vi "导出文件流程.vi"(0 "刷新错误?":refnum<vi>, 1 "刷新信号-引用":refnum<vi>, 2 "XY图更新错误?":refnum<vi>, 3 "XY图-引用":refnum<vi>, 6 "错误输入":errorcluster, 7 "查询界面VI-引用":refnum<vi>, 8 "累积记录-引用":refnum<vi>, 9 "设备清单-引用":refnum<vi>, 10 "设备列表-引用":refnum<vi>, 11 "导出条件":T2) -> (4 "错误输出":errorcluster)   [LabVIEW 2017]
uses:
  e6222c88-c07e-4ecc-8f52-69902710a8a5.vi
  642c5d25-862a-469e-85c1-2600a8577a38.vi
  <vilib>/Utility/file.llb/Write Delimited Spreadsheet (string).vi
panel:
  in  "刷新次数":i32
  in  "原界面模式":T1
  out "提示语":string
  # "导出记录执行中......"
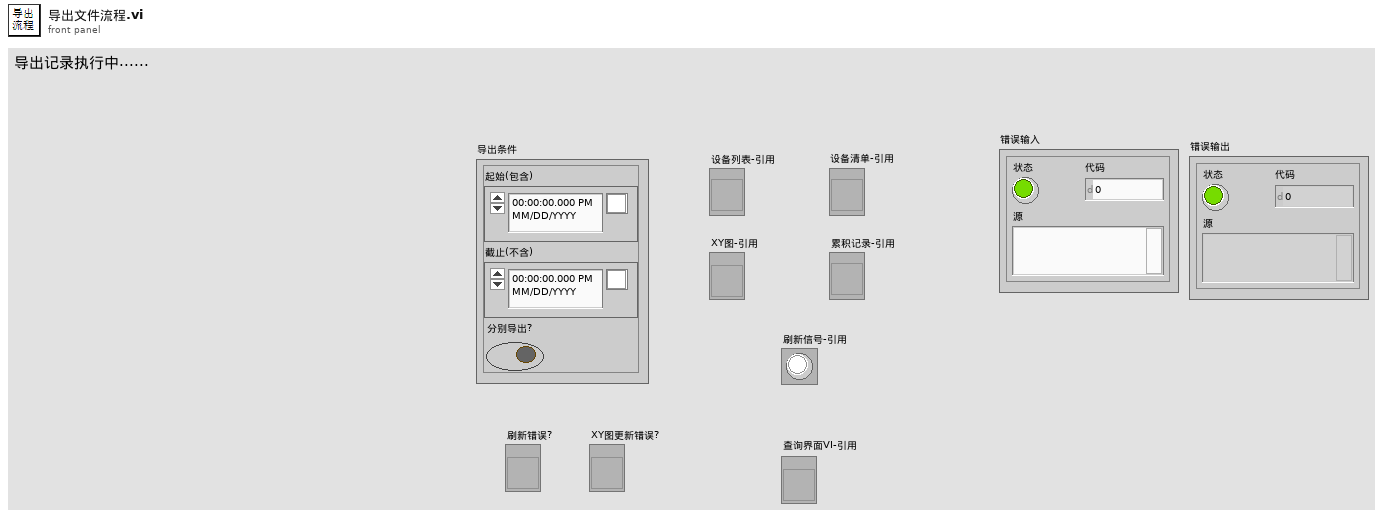
[diagram p1: front panel]
types:
  T1 = typedef "枚举-顶层框架功能模式.ctl" = enum16{"管理模式", "监测模式", "浏览模式"}
  T2 = typedef "文件导出条件.ctl" = cluster{"起始(包含)":timestamp, "截止(不含)":timestamp, "分别导出?":bool}
  T3 = typedef "定时配置.ctl" = cluster{"定时模式":enum16{"绝对时间", "相对时间"}, "单位":enum16{"年", "月", "日", "时", "分"}, "间隔":u8, "目标时刻":timestamp}
  T4 = enum32{"Invalid", "Standard", "Closed", "Hidden", "Minimized", "Maximized"}
  T5 = typedef "探测器信息.ctl" = cluster{"网络地址":string, "名称":string, "备注":string, "累积剂量":dbl, "累积限值":dbl, "硬件剂量率限值":T6, "剂量率限值1":dbl, "剂量率限值2":dbl, "报警方式":T7}
  T6 = typedef "探头剂量率限值选择.ctl" = enum16{"一级限值", "二级限值"}
  T7 = typedef "报警方式选择.ctl" = enum16{"常报警", "自动静音", "手动静音"}
  T8 = typedef "单条累积记录.ctl" = cluster{"起始时间":timestamp, "结束时间":timestamp, "累积剂量":dbl}
  T9 = typedef "通用报警记录.ctl" = cluster{"探头状态":T10, "探头地址与信息":T5, "缓存绘图数据":T11, "平均值":dbl, "报警时长":cluster{"分":u16, "秒":u16}, "结论":string}
  T10 = typedef "探头状态.ctl" = enum16{"正常", "离线", "禁用", "一级报警", "二级报警", "累积报警"}
  T11 = typedef "缓存数据.ctl" = cluster{"时间":timestamp[], "数值":dbl[], "压缩等级数量":i32[], "最大值":cluster{"时间":timestamp, "数值":dbl}, "起始点":cluster{"时间":timestamp, "数值":dbl}, "容量限值":i32, "报警累积":dbl}
  T12 = cluster{"累积曲线数据":T8[], "累积列表内容":string[], "匹配的报警数据":cluster{"名称":string, "路径":path, "内容":string, "报警记录":T9}[]}[]
  T13 = typedef "imagedata.ctl" = cluster{"image type":i32, "image depth":i32, "image":u8[], "mask":u8[], "colors":u32[], "Rectangle":cluster{"left":i16, "top":i16, "right":i16, "bottom":i16}}
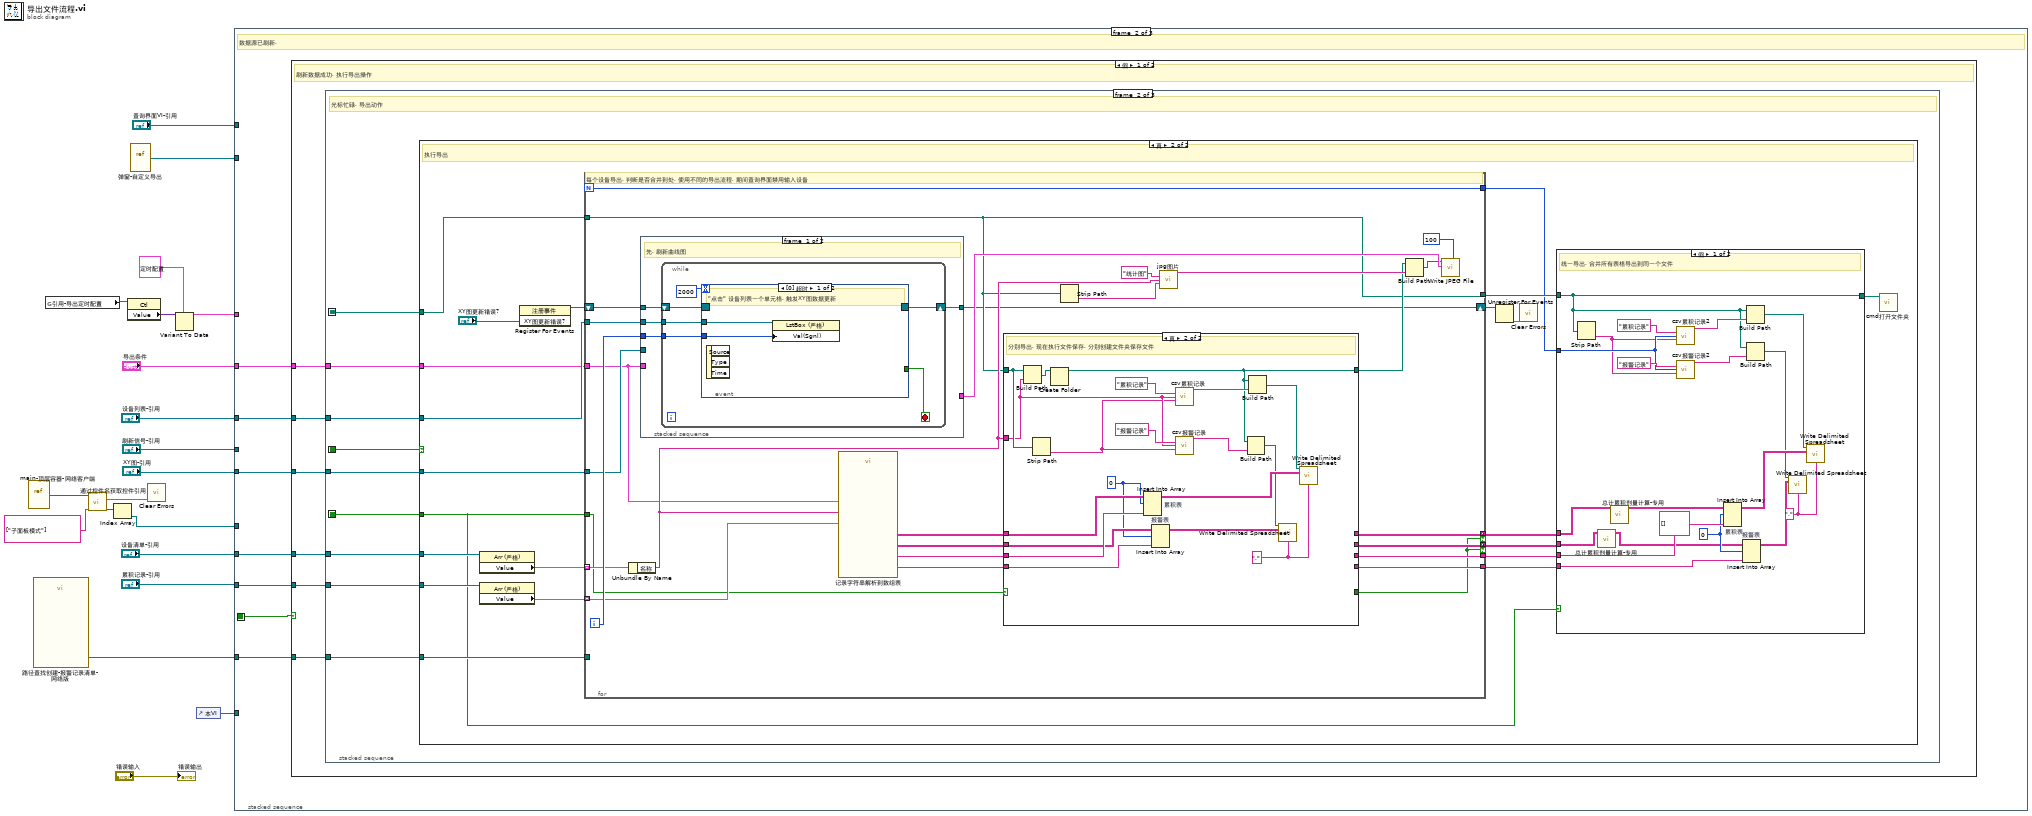
[diagram p0: block diagram]
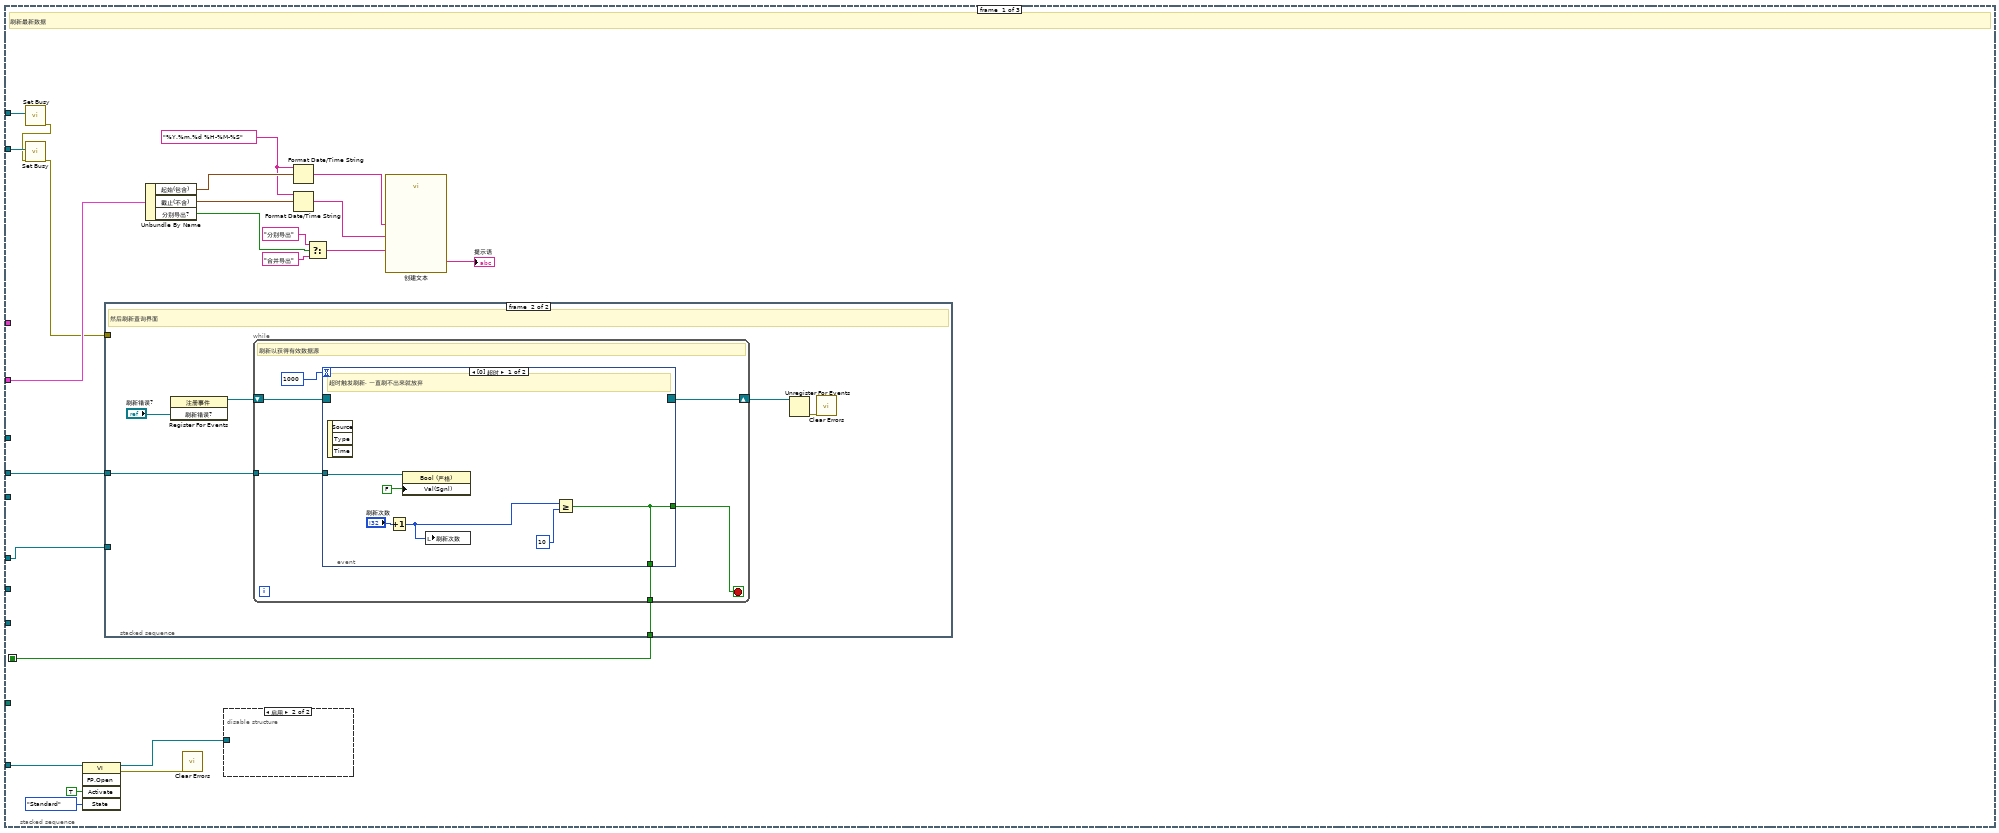
[diagram p2: hidden frame]
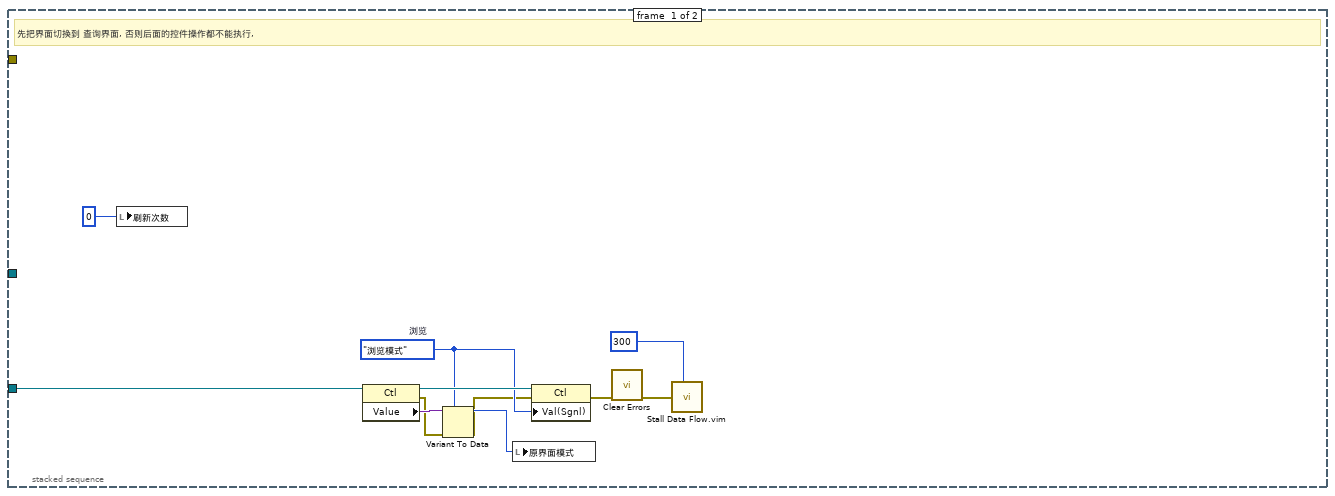
[diagram p3: hidden frame]
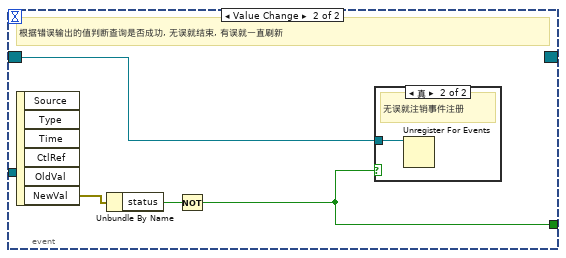
[diagram p4: hidden frame]
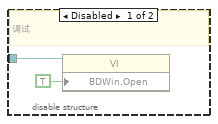
[diagram p6: hidden frame]
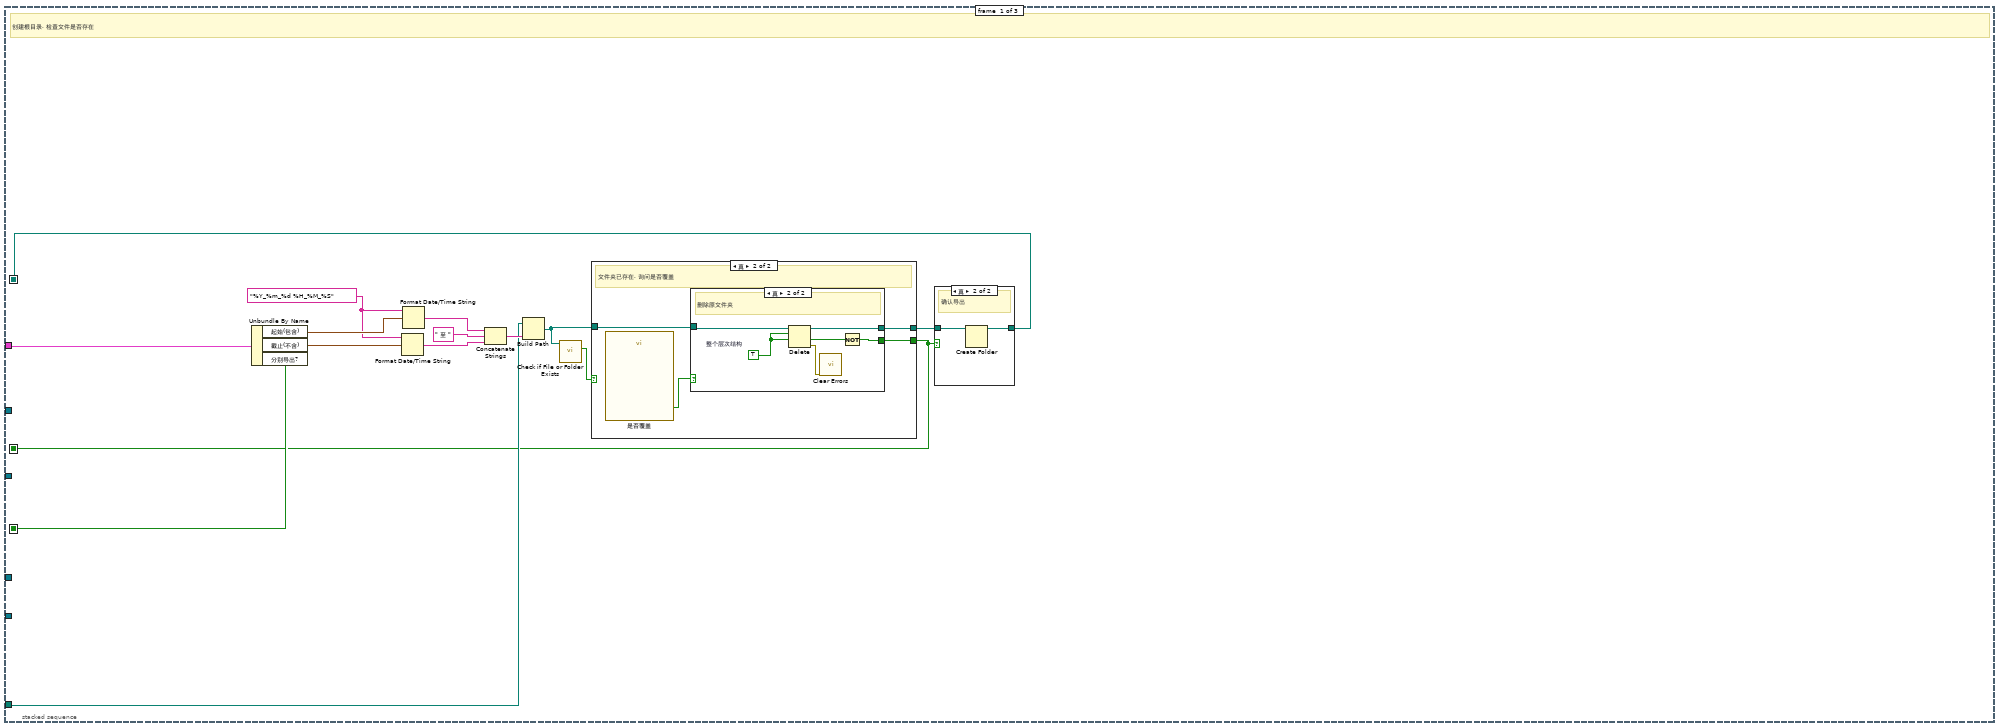
[diagram p7: hidden frame]
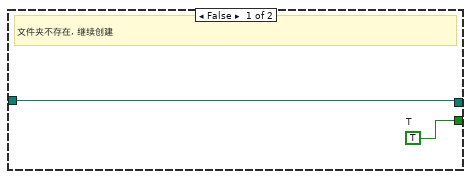
[diagram p8: hidden frame]
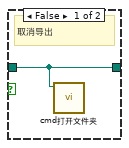
[diagram p10: hidden frame]
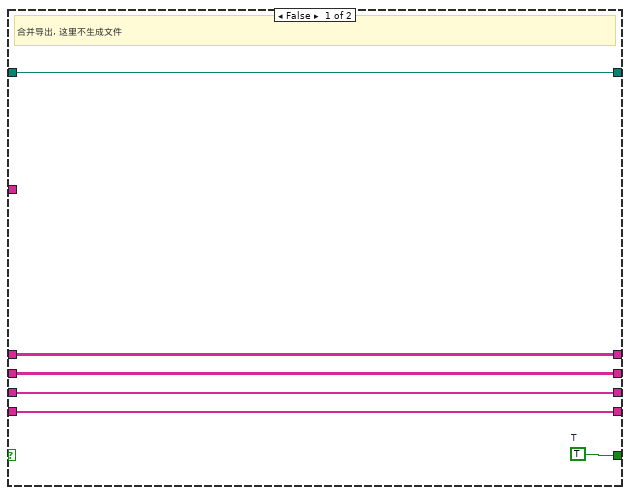
[diagram p13: hidden frame]
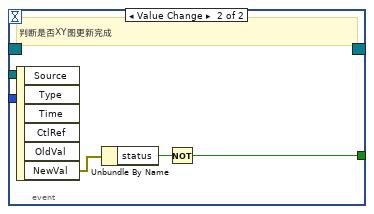
[diagram p14: hidden frame]
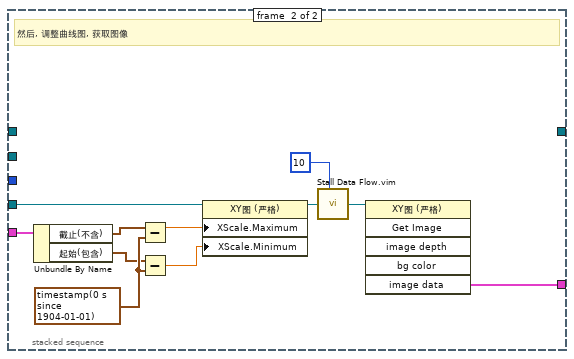
[diagram p15: hidden frame]
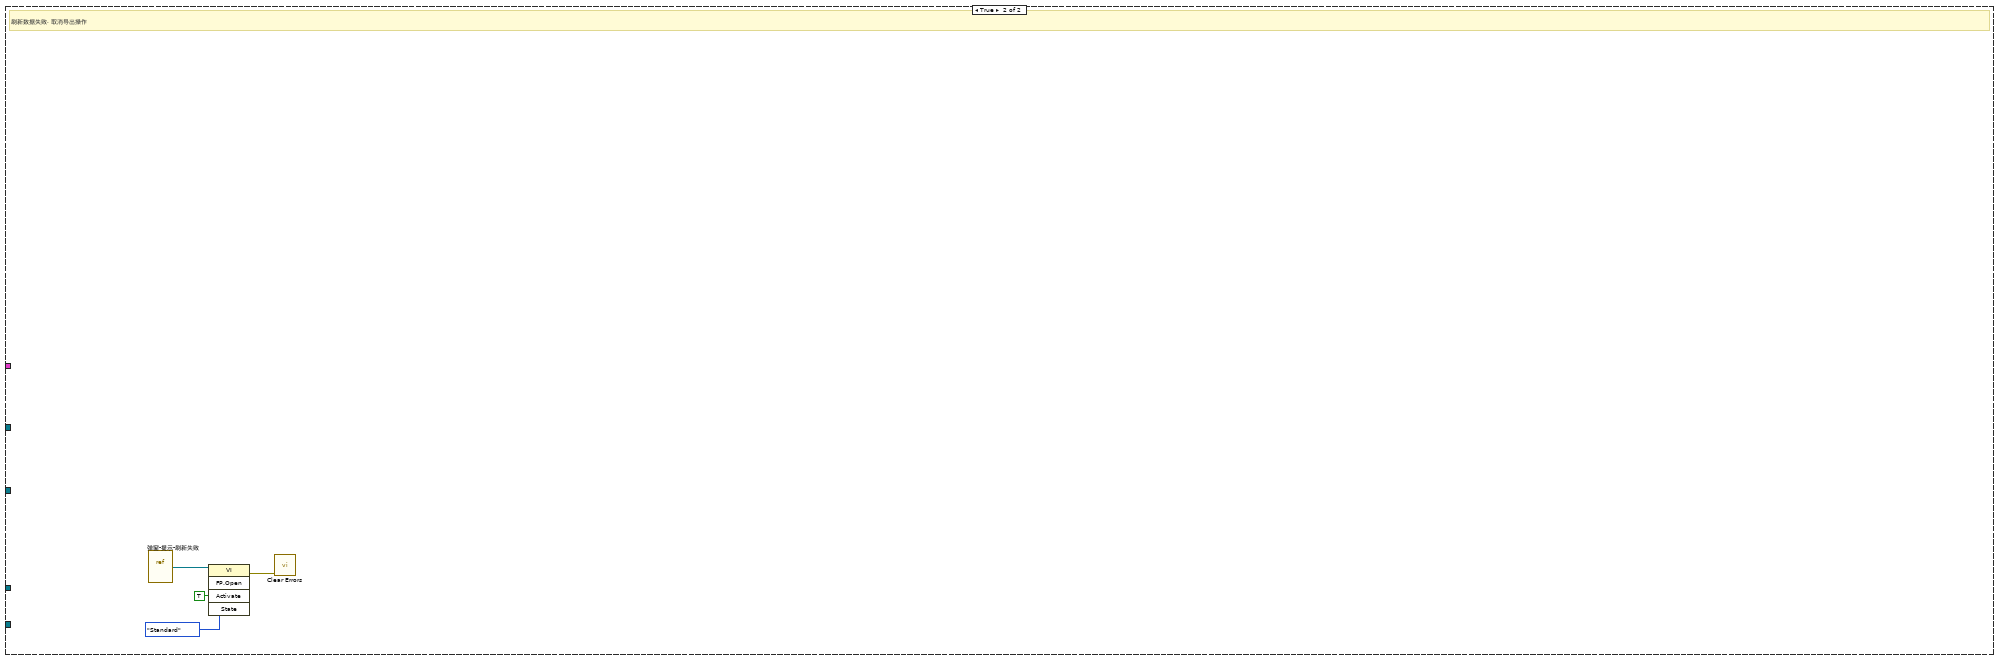
[diagram p17: hidden frame]
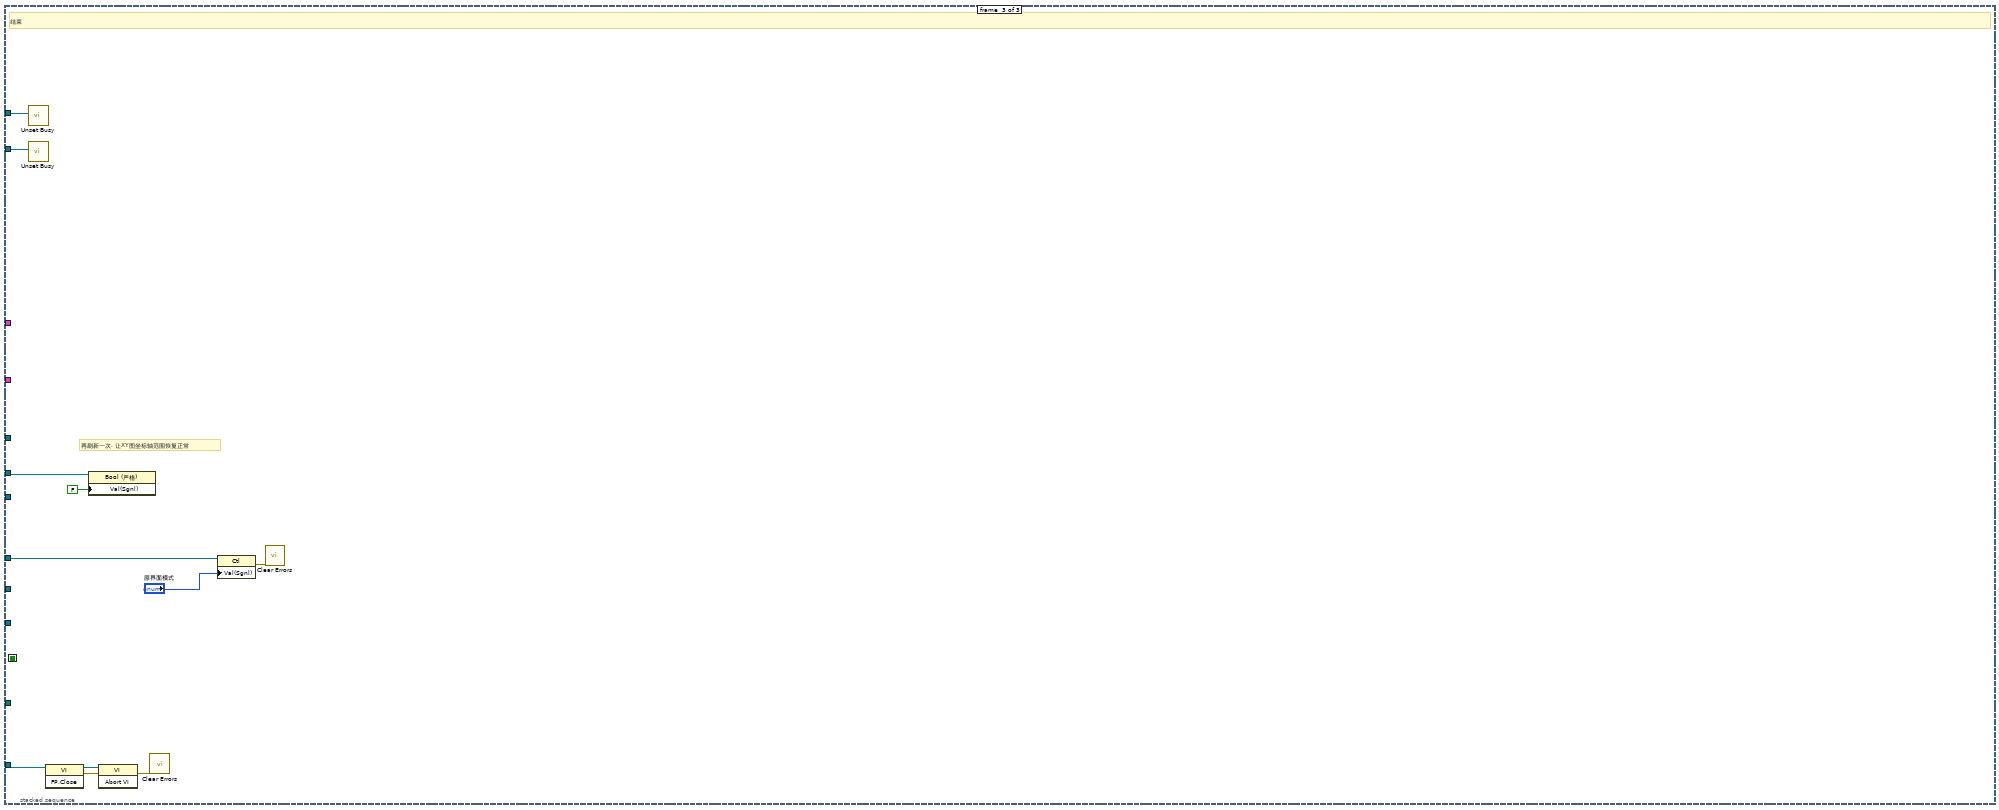
[diagram p18: hidden frame]
diagram:
  n1 = vi-ref "main-顶层容器-网络客户端.vi"() -> (w6:refnum<vi>)
  n2 = call "路径查找创建-报警记录清单-网络版.vi"() -> ("导出记录"=w11:path)  [unwired: 2 in, 13 out]
  n3 = global read "全局变量-35点监测.vi" "引用-导出定时配置"() -> (w15:refnum<vi>)
  n4 = call "通过控件名获取控件引用.vi"("控件名数组"=string[] ["子面板模式"], "VI引用"=w6) -> ("控件引用输出"=w5:refnum<vi>[], "错误输出"=w2:errorcluster)  [unwired: 7 in, 1 out]
  n5 = Index Array(array=w5) -> (element=w3:refnum<vi>)  [unwired: 1 in]
  n6 = property class="Ctl"(reference=w15) -> ("Value"=w14:variant)  [unwired: 1 in, 2 out]
  n7 = vi-ref "弹窗-自定义导出.vi"() -> (w1:refnum<vi>)
  n8 = call <vilib>:"Clear Errors.vi"("error in (no error)"=w2) -> ()  [unwired: 5 in, 2 out]
  n9 = Variant To Data(type=T3 {"定时模式"=enum."绝对时间", "单位"=enum."年", "间隔"=0, "目标时刻"=timestamp(0 s since 1904-01-01)} ("定时配置"), Variant=w14) -> (data=w12:T3)  [unwired: 1 in, 1 out]
  n10 = control-ref of="本VI"() -> (w8:refnum<vi>)
  n11 = stacked-sequence {
    seq-local: [w26 _ _] -> [_ w80 _]
    tunnel: "设备列表-引用" -> [_ w84 _]
    tunnel: "刷新信号-引用" -> [w43 _ w262]
    tunnel: "XY图-引用" -> [_ w85 _]
    tunnel: "设备清单-引用" -> [_ w86 _]
    tunnel: "累积记录-引用" -> [_ w83 _]
    tunnel: "导出条件" -> [w42 w82 _]
    tunnel: w12 -> [_ _ _]
    tunnel: w11 -> [_ w81 _]
    tunnel: w8 -> [w31 _ w267]
    tunnel: "查询界面VI-引用" -> [w25 _ w259]
    tunnel: w3 -> [w24 _ w258]
    tunnel: w1 -> [w23 _ w257]
    frame #0 {
      w39 = "%Y.%m.%d %H-%M-%S" ("时间格式字符串(%c)")
      # "刷新最新数据"
      n12 = call <vilib>:"Set Busy.vi"("VI reference (current VI)"=w25) -> ("error out"=w22:errorcluster)  [unwired: 9 in, 1 out]
      n13 = call <vilib>:"Set Busy.vi"("error in (no error)"=w22, "VI reference (current VI)"=w23) -> ("error out"=w21:errorcluster)  [unwired: 8 in, 1 out]
      n14 = invoke class="VI" method="FP.Open"(reference=w31, "Activate"=TRUE ("激活？"), "State"=T4."Standard" ("状态")) -> (reference out=w27:refnum<vi>, error out=w28:errorcluster)  [unwired: 2 in, 3 out]
      n15 = stacked-sequence {
        tunnel: w43 -> [_ w57]
        tunnel: [_ w55] -> w26
        tunnel: w21 -> [_ _]
        tunnel: w24 -> [w44 _]
        frame #0 {
          w51 = 枚举-顶层框架功能模式."浏览模式"  # 浏览
          # "先把界面切换到 查询界面, 否则后面的控件操作都不能执行,"
          n16 = local write "刷新次数"(0 ("数值输入控件")) -> ()
          n17 = property class="Ctl"(reference=w44) -> (reference out=w53:refnum<vi>, error out=w47:errorcluster, "Value"=w52:variant)  [unwired: 1 in]
          n18 = Variant To Data(error in=w47, type=w51, Variant=w52) -> (data=w50:T1, error out=w46:errorcluster)
          n19 = local write "原界面模式"(w50) -> ()
          n20 = property class="Ctl"(reference=w53, error in=w46, "Val(Sgnl)"=w51) -> (error out=w54:errorcluster)  [unwired: 1 out]
          n21 = call <vilib>:"Clear Errors.vi"("error in (no error)"=w54) -> ("error out"=w49:errorcluster)  [unwired: 5 in, 1 out]
          n22 = call "Stall Data Flow.vim"("value in"=w49, "milliseconds to wait"=u32 300) -> ()  [unwired: 2 out]
        }
        frame #1 {
          # "然后刷新查询界面"
          n23 = register-events("刷新错误?") -> (reference out=w59:refnum<event-registration>)  [unwired: 2 in, 1 out]
          n24 = while {
            tunnel: w57 -> [w63]
            shift-right: [w62] -> w56
            shift-left: w59 -> [w66]
            tunnel: [w61] -> w55
            stop <- w64 stop-if-true
            # "刷新以获得有效数据源"
            n25 = event shown="[0] 超时" {
              selector: w66 -> [_ w74]
              dyn-events: [_ _] -> w62
              timeout: 1000 -> [_ _]
              tunnel: [w69 w73] -> w64
              tunnel: w63 -> [w72 _]
              tunnel: [w69 _] -> w61
              event Timeout {
                # "超时触发刷新, 一直刷不出来就放弃"
                n26 = event-data() -> ()  [unwired: 1 in, 3 out]
                n27 = Increment(x="刷新次数") -> (x+1=w67:i32)
                n28 = property class="Bool (严格)"(reference=w72, "Val(Sgnl)"=FALSE) -> ()  [unwired: 1 in, 2 out]
                n29 = local write "刷新次数"(w67) -> ()
                n30 = Greater Or Equal?(x=w67, y=10) -> (x >= y?=w69:bool)
              }
              event Value Change {
                # "根据错误输出的值判断查询是否成功, 无误就结束, 有误就一直刷新"
                n31 = event-data() -> ("NewVal"=w76:errorcluster)  [unwired: 1 in, 5 out]
                n32 = Unbundle By Name(w76) -> ("status"=w75:bool)
                n33 = Not(x=w75) -> (.not. x?=w73:bool)
                n34 = case shown="真" w73 {
                  tunnel: w74 -> [_ w77]
                  frame False {
                  }
                  frame True {
                    # "无误就注销事件注册"
                    n35 = Unregister For Events(event registration refnum=w77) -> ()  [unwired: 1 in, 1 out]
                  }
                }
              }
            }
          }
          n36 = Unregister For Events(event registration refnum=w56) -> (error out=w58:errorcluster)  [unwired: 1 in]
          n37 = call <vilib>:"Clear Errors.vi"("error in (no error)"=w58) -> ()  [unwired: 5 in, 2 out]
        }
      }
      n38 = Unbundle By Name(w42) -> ("起始(包含)"=w41:timestamp, "截止(不含)"=w40:timestamp, "分别导出?"=w34:bool)
      n39 = call <vilib>:"Clear Errors.vi"("error in (no error)"=w28) -> ()  [unwired: 5 in, 2 out]
      n40 = disable-structure shown="启用" {
        disable-tunnel: w27 -> [w78 _]
        frame Disabled {
          # "调试"
          n41 = property class="VI"(reference=w78, "BDWin.Open"=TRUE ("程序框图窗口:打开")) -> ()  [unwired: 1 in, 2 out]
        }
        frame Enabled {
        }
      }
      n42 = Format Date/Time String(time format string (%c)=w39, seconds (now)=w40) -> (date/time string=w37:string)  [unwired: 1 in]
      n43 = Format Date/Time String(time format string (%c)=w39, seconds (now)=w41) -> (date/time string=w38:string)  [unwired: 1 in]
      n44 = Select(t="分别导出", s=w34, f="合并导出") -> (s? t:f=w33:string)
      n45 = call "创建文本"("起始"=w38, "截止"=w37, "导出模式"=w33) -> ("Result"=→"提示语":string)  [unwired: 11 in, 1 out]
    }
    frame #1 {
      # "数据源已刷新,"
      n46 = case shown="假" w80 {
        tunnel: w86 -> [w92 _]
        tunnel: w85 -> [w91 _]
        tunnel: w84 -> [w90 _]
        tunnel: w83 -> [w89 _]
        tunnel: w82 -> [w88 _]
        tunnel: w81 -> [w87 _]
        frame False {
          # "刷新数据成功, 执行导出操作"
          n47 = stacked-sequence {
            seq-local: [w99 _ _] -> [_ w126 _]
            seq-local: [w97 _ _] -> [_ w125 _]
            seq-local: [w94 _ _] -> [_ w124 _]
            tunnel: w92 -> [_ w132 _]
            tunnel: w91 -> [_ w131 _]
            tunnel: w90 -> [_ w130 _]
            tunnel: w88 -> [w100 w127 _]
            tunnel: w89 -> [_ w129 _]
            tunnel: w87 -> [w98 w128 _]
            frame #0 {
              w101 = "%Y_%m_%d %H_%M_%S" ("时间格式字符串(%c)")
              # "创建根目录, 检查文件是否存在"
              n48 = Unbundle By Name(w100) -> ("起始(包含)"=w105:timestamp, "截止(不含)"=w106:timestamp, "分别导出?"=w97:bool)
              n49 = Format Date/Time String(time format string (%c)=w101, seconds (now)=w106) -> (date/time string=w104:string)  [unwired: 1 in]
              n50 = Format Date/Time String(time format string (%c)=w101, seconds (now)=w105) -> (date/time string=w103:string)  [unwired: 1 in]
              n51 = Concatenate Strings(w103, " 至 " ("字符串"), w104) -> (w107:string)
              n52 = Build Path(base path=w98, name or relative path=w107) -> (appended path=w96:path)
              n53 = call <vilib>:"Check if File or Folder Exists.vi"("path"=w96) -> ("file or folder exists?"=w93:bool)  [unwired: 8 in, 2 out]
              n54 = case shown="真" w93 {
                tunnel: w96 -> [w108 w112]
                tunnel: [w108 w111] -> w95
                tunnel: [w109 w110] -> w94
                frame False {
                  w109 = TRUE  # T
                  # "文件夹不存在, 继续创建"
                }
                frame True {
                  # "文件夹已存在, 询问是否覆盖"
                  n55 = call "是否覆盖"() -> ("覆盖"=w113:bool)  [unwired: 10 in, 1 out]
                  n56 = case shown="真" w113 {
                    tunnel: w112 -> [w114 w120]
                    tunnel: [w114 w119] -> w111
                    tunnel: [_ w115] -> w110
                    frame False {
                      # "取消导出"
                    }
                    frame True {
                      w118 = TRUE  # 整个层次结构
                      # "删除原文件夹"
                      n57 = Delete(path (use dialog)=w120, entire hierarchy (F)=w118, confirm (F)=w118) -> (deleted path=w119:path, cancelled=w116:bool, error out=w117:errorcluster)  [unwired: 2 in]
                      n58 = call <vilib>:"Clear Errors.vi"("error in (no error)"=w117) -> ()  [unwired: 5 in, 2 out]
                      n59 = Not(x=w116) -> (.not. x?=w115:bool)
                    }
                  }
                }
              }
              n60 = case shown="真" w94 {
                tunnel: [w121 w123] -> w99
                tunnel: w95 -> [w121 w122]
                frame False {
                  # "取消导出"
                  n61 = call "cmd打开文件夹.vi"("文件路径"=w121) -> ()  [unwired: 10 in, 1 out]
                }
                frame True {
                  # "确认导出"
                  n62 = Create Folder(path (use dialog)=w122) -> (created path=w123:path)  [unwired: 2 in, 2 out]
                }
              }
            }
            frame #1 {
              # "光标忙碌, 导出动作"
              n63 = case shown="真" w124 {
                tunnel: w132 -> [_ w153]
                tunnel: w131 -> [_ w151]
                tunnel: w130 -> [_ w148]
                tunnel: w129 -> [_ w147]
                tunnel: w128 -> [_ w145]
                tunnel: w127 -> [_ w138]
                tunnel: w126 -> [_ w137]
                tunnel: w125 -> [_ w136]
                frame False {
                  # "取消导出"
                }
                frame True {
                  # "执行导出"
                  n64 = property class="Arr (严格)"(reference=w153) -> ("Value"=w152:T5[])  [unwired: 1 in, 2 out]
                  n65 = property class="Arr (严格)"(reference=w147) -> ("Value"=w146:T12)  [unwired: 1 in, 2 out]
                  n66 = register-events("XY图更新错误?") -> (reference out=w149:refnum<event-registration>)  [unwired: 2 in, 1 out]
                  n67 = for {
                    N -> [w187]
                    tunnel: w152 -> [w197] mode=indexing
                    tunnel: w151 -> [w198]
                    tunnel: w148 -> [w200]
                    tunnel: w138 -> [w176]
                    tunnel: w146 -> [w196] mode=indexing
                    tunnel: w145 -> [_]
                    tunnel: w137 -> [w179]
                    tunnel: [w191] -> w144 mode=concatenating if=w185
                    tunnel: [w190] -> w142 mode=concatenating if=w185
                    tunnel: [w189] -> w143
                    tunnel: [w188] -> w141
                    tunnel: [w179] -> w140
                    tunnel: [w187] -> w139
                    tunnel: w136 -> [w177]
                    shift-right: [w175] -> w135
                    shift-left: w149 -> [w201]
                    i -> [w199]
                    # "每个设备导出, 判断是否合并到处, 使用不同的导出流程, 期间查询界面禁用输入设备"
                    n68 = Unbundle By Name(w197) -> ("名称"=w180:string)
                    n69 = stacked-sequence {
                      tunnel: w201 -> [w230 _]
                      tunnel: w200 -> [w229 _]
                      tunnel: w199 -> [w228 _]
                      tunnel: w198 -> [_ w252]
                      tunnel: w176 -> [_ w251]
                      tunnel: [_ w244] -> w186
                      tunnel: [w227 _] -> w175
                      frame #0 {
                        # "先, 刷新曲线图"
                        n70 = while {
                          tunnel: w229 -> [w234]
                          tunnel: w228 -> [w233]
                          shift-right: [w231] -> w227
                          shift-left: w230 -> [w236]
                          stop <- w232 stop-if-true
                          n71 = event shown="[0] 超时" {
                            selector: w236 -> [_ _]
                            dyn-events: [_ _] -> w231
                            timeout: 2000 -> [_ _]
                            tunnel: w234 -> [w237 _]
                            tunnel: w233 -> [w238 _]
                            tunnel: [_ w239] -> w232
                            event Timeout {
                              # "\"点击\" 设备列表一个单元格, 触发XY图数据更新"
                              n72 = event-data() -> ()  [unwired: 1 in, 3 out]
                              n73 = property class="LstBox (严格)"(reference=w237, "Val(Sgnl)"=w238) -> ()  [unwired: 1 in, 2 out]
                            }
                            event Value Change {
                              # "判断是否XY图更新完成"
                              n74 = event-data() -> ("NewVal"=w241:errorcluster)  [unwired: 1 in, 5 out]
                              n75 = Unbundle By Name(w241) -> ("status"=w240:bool)
                              n76 = Not(x=w240) -> (.not. x?=w239:bool)
                            }
                          }
                        }
                      }
                      frame #1 {
                        w248 = timestamp(0 s since 1904-01-01)
                        # "然后, 调整曲线图, 获取图像"
                        n77 = Unbundle By Name(w251) -> ("截止(不含)"=w250:timestamp, "起始(包含)"=w247:timestamp)
                        n78 = Subtract(x=w250, y=w248) -> (x-y=w249:dbl)
                        n79 = Subtract(x=w247, y=w248) -> (x-y=w246:dbl)
                        n80 = property class="XY图 (严格)"(reference=w252, "XScale.Maximum"=w249, "XScale.Minimum"=w246) -> (reference out=w245:refnum<vi>)  [unwired: 1 in, 1 out]
                        n81 = call "Stall Data Flow.vim"("value in"=w245, "milliseconds to wait"=u32 10) -> ("value out"=w243:refnum<vi>)  [unwired: 1 out]
                        n82 = invoke class="XY图 (严格)" method="Get Image"(reference=w243) -> ("image data"=w244:T13)  [unwired: 5 in, 5 out]
                      }
                    }
                    n83 = call "记录字符串解析到数组表.vi"("导出条件"=w176, "记录数据"=w196, "名称"=w180) -> ("累积列表-标题行"=w193:string[], "报警列表-标题行"=w192:string[], "报警列表数组"=w194:string[][], "累积记录数组"=w195:string[][])  [unwired: 5 in]
                    n84 = case shown="真" w177 {
                      tunnel: w179 -> [w202 w212]
                      tunnel: w195 -> [w207 w226]
                      tunnel: w194 -> [w206 w224]
                      tunnel: w193 -> [w205 w225]
                      tunnel: w192 -> [w204 w223]
                      tunnel: w180 -> [_ w211]
                      tunnel: [w207 _] -> w191
                      tunnel: [w206 _] -> w190
                      tunnel: [w205 _] -> w189
                      tunnel: [w204 _] -> w188
                      tunnel: [w203 _] -> w185
                      tunnel: [w202 w210] -> w181
                      frame False {
                        w203 = TRUE  # T
                        # "合并导出, 这里不生成文件"
                      }
                      frame True {
                        w208 = 0 ("索引 (行)")
                        w220 = "," ("delimiter (\\t)")
                        # "分别导出, 现在执行文件保存, 分别创建文件夹保存文件"
                        n85 = Build Path(base path=w212, name or relative path=w211) -> (appended path=w213:path)
                        n86 = Strip Path(path=w212) -> (name=w209:string)  [unwired: 1 out]
                        n87 = Create Folder(path (use dialog)=w213) -> (created path=w210:path)  [unwired: 2 in, 2 out]
                        n88 = Insert Into Array "累积表"(array=w226, index (row)=w208, new element=w225) -> (w222:string[][])  [unwired: 1 in]
                        n89 = Insert Into Array "报警表"(array=w224, index (row)=w208, new element=w223) -> (w221:string[][])  [unwired: 1 in]
                        n90 = call "csv累积记录"("文件类型"="累积记录", "名称"=w211, "日期"=w209) -> ("Result"=w217:string)  [unwired: 11 in, 1 out]
                        n91 = call "csv报警记录"("文件类型"="报警记录", "名称"=w211, "日期"=w209) -> ("Result"=w216:string)  [unwired: 11 in, 1 out]
                        n92 = Build Path(base path=w210, name or relative path=w216) -> (appended path=w214:path)
                        n93 = Build Path(base path=w210, name or relative path=w217) -> (appended path=w215:path)
                        n94 = call-poly <vilib>:"Write Delimited Spreadsheet.vi"("file path (dialog if empty)"=w214, "2D data"=w221, "delimiter (\\t)"=w220) -> ()  [unwired: 11 in, 2 out]
                        n95 = call-poly <vilib>:"Write Delimited Spreadsheet.vi"("file path (dialog if empty)"=w215, "2D data"=w222, "delimiter (\\t)"=w220) -> ()  [unwired: 11 in, 2 out]
                      }
                    }
                    n96 = Strip Path(path=w179) -> (name=w174:string)  [unwired: 1 out]
                    n97 = call "jpg图片"("文件类型"="统计图", "名称"=w180, "日期"=w174) -> ("Result"=w183:string)  [unwired: 11 in, 1 out]
                    n98 = Build Path(base path=w181, name or relative path=w183) -> (appended path=w178:path)
                    n99 = call <vilib>:"Write JPEG File.vi"("quality (80)"=100, "image data"=w186, "path to JPEG file"=w178) -> ()  [unwired: 7 in, 2 out]
                  }
                  n100 = Unregister For Events(event registration refnum=w135) -> (error out=w134:errorcluster)  [unwired: 1 in]
                  n101 = call <vilib>:"Clear Errors.vi"("error in (no error)"=w134) -> ()  [unwired: 5 in, 2 out]
                  n102 = case shown="假" w136 {
                    tunnel: w144 -> [w157 _]
                    tunnel: w143 -> [w172 _]
                    tunnel: w142 -> [w155 _]
                    tunnel: w141 -> [w171 _]
                    tunnel: w140 -> [w158 w173]
                    tunnel: w139 -> [w166 _]
                    tunnel: [w158 w173] -> w133
                    frame False {
                      (unwired) string[][] [] ("累积记录数组")
                      w159 = 0 ("索引 (行)")
                      w165 = "," ("delimiter (\\t)")
                      # "统一导出, 合并所有表格导出到同一个文件"
                      n103 = Strip Path(path=w158) -> (name=w160:string)  [unwired: 1 out]
                      n104 = call "总计累积剂量计算-专用.vi"("记录数组"=w155) -> ("输出记录数组"=w154:string[][])  [unwired: 10 in]
                      n105 = call "总计累积剂量计算-专用.vi"("记录数组"=w157) -> ("输出记录数组"=w156:string[][])  [unwired: 10 in]
                      n106 = call "csv累积记录2"("文件类型"="累积记录", "数量"=w166, "日期"=w160) -> ("Result"=w169:string)  [unwired: 11 in, 1 out]
                      n107 = call "csv报警记录2"("文件类型"="报警记录", "数量"=w166, "日期"=w160) -> ("Result"=w170:string)  [unwired: 11 in, 1 out]
                      n108 = Insert Into Array "累积表"(array=w156, index (row)=w159, new element=w172) -> (w164:string[][])  [unwired: 1 in]
                      n109 = Insert Into Array "报警表"(array=w154, index (row)=w159, new element=w171) -> (w163:string[][])  [unwired: 1 in]
                      n110 = Build Path(base path=w158, name or relative path=w169) -> (appended path=w162:path)
                      n111 = Build Path(base path=w158, name or relative path=w170) -> (appended path=w161:path)
                      n112 = call-poly <vilib>:"Write Delimited Spreadsheet.vi"("file path (dialog if empty)"=w161, "2D data"=w163, "delimiter (\\t)"=w165) -> ()  [unwired: 11 in, 2 out]
                      n113 = call-poly <vilib>:"Write Delimited Spreadsheet.vi"("file path (dialog if empty)"=w162, "2D data"=w164, "delimiter (\\t)"=w165) -> ()  [unwired: 11 in, 2 out]
                    }
                    frame True {
                      # "分别导出, 此处不执行"
                    }
                  }
                  n114 = call "cmd打开文件夹.vi"("文件路径"=w133) -> ()  [unwired: 10 in, 1 out]
                }
              }
            }
            frame #2 {
              # "取消忙碌光标"
            }
          }
        }
        frame True {
          # "刷新数据失败, 取消导出操作"
          n115 = vi-ref "弹窗-提示-刷新失败.vi"() -> (w254:refnum<vi>)
          n116 = invoke class="VI" method="FP.Open"(reference=w254, "Activate"=TRUE ("激活？"), "State"=T4."Standard" ("状态")) -> (error out=w253:errorcluster)  [unwired: 2 in, 4 out]
          n117 = call <vilib>:"Clear Errors.vi"("error in (no error)"=w253) -> ()  [unwired: 5 in, 2 out]
        }
      }
    }
    frame #2 {
      # "再刷新一次, 让XY图坐标轴范围恢复正常"
      # "结束"
      n118 = call <vilib>:"Unset Busy.vi"("VI reference (current VI)"=w259) -> ()  [unwired: 10 in, 1 out]
      n119 = call <vilib>:"Unset Busy.vi"("VI reference (current VI)"=w257) -> ()  [unwired: 10 in, 1 out]
      n120 = invoke class="VI" method="FP.Close"(reference=w267) -> (reference out=w266:refnum<vi>, error out=w265:errorcluster)  [unwired: 2 in, 1 out]
      n121 = property class="Bool (严格)"(reference=w262, "Val(Sgnl)"=FALSE) -> ()  [unwired: 1 in, 2 out]
      n122 = invoke class="VI" method="Abort VI"(reference=w266, error in=w265) -> (error out=w264:errorcluster)  [unwired: 1 in, 2 out]
      n123 = call <vilib>:"Clear Errors.vi"("error in (no error)"=w264) -> ()  [unwired: 5 in, 2 out]
      n124 = property class="Ctl"(reference=w258, "Val(Sgnl)"="原界面模式") -> (error out=w261:errorcluster)  [unwired: 1 in, 1 out]
      n125 = call <vilib>:"Clear Errors.vi"("error in (no error)"=w261) -> ()  [unwired: 5 in, 2 out]
    }
  }
  "错误输出" <- "错误输入"
